vi "浊度电极校准.vi"() -> ()   [LabVIEW 2016, in "斯坦道多参数.lvlib"]
uses:
  <vilib>/Utility/miscctls.llb/LVPointTypeDef.ctl
  <vilib>/Analysis/NI_AALBase.lvlib
panel:
  out "第二点校准值":dbl
  out "第一点校准值":dbl
  in  "校准停止":bool
  in  "校准启动":bool
  in  "校准模式":enum16{"两点校准", "单点校准"}(ring)
  out "最小值":sgl format="%#.2f"
  out "最大值":sgl format="%#.2f"
  out "波形图表":sgl(graph) caption="历史曲线"
  out "mean":dbl caption="均值" format="%#.2f"
  out "standard deviation":dbl caption="标准差" format="%#.2f"
  out "变异系数":dbl format="%#.6f"
  out "测量值":dbl
  out "提示":string
  out "标液2":dbl
  out "标液1":dbl
  out "原始读取值":dbl caption="信号值"
  out "偏移值补偿":dbl
  out "电极斜率":dbl
  out "电极零点":dbl
  # "浊度电极设定"
  # "NTU"
  # "%"
  # "NTU"
  # "NTU"
  # "NTU"
  # "请选择校准模式:"
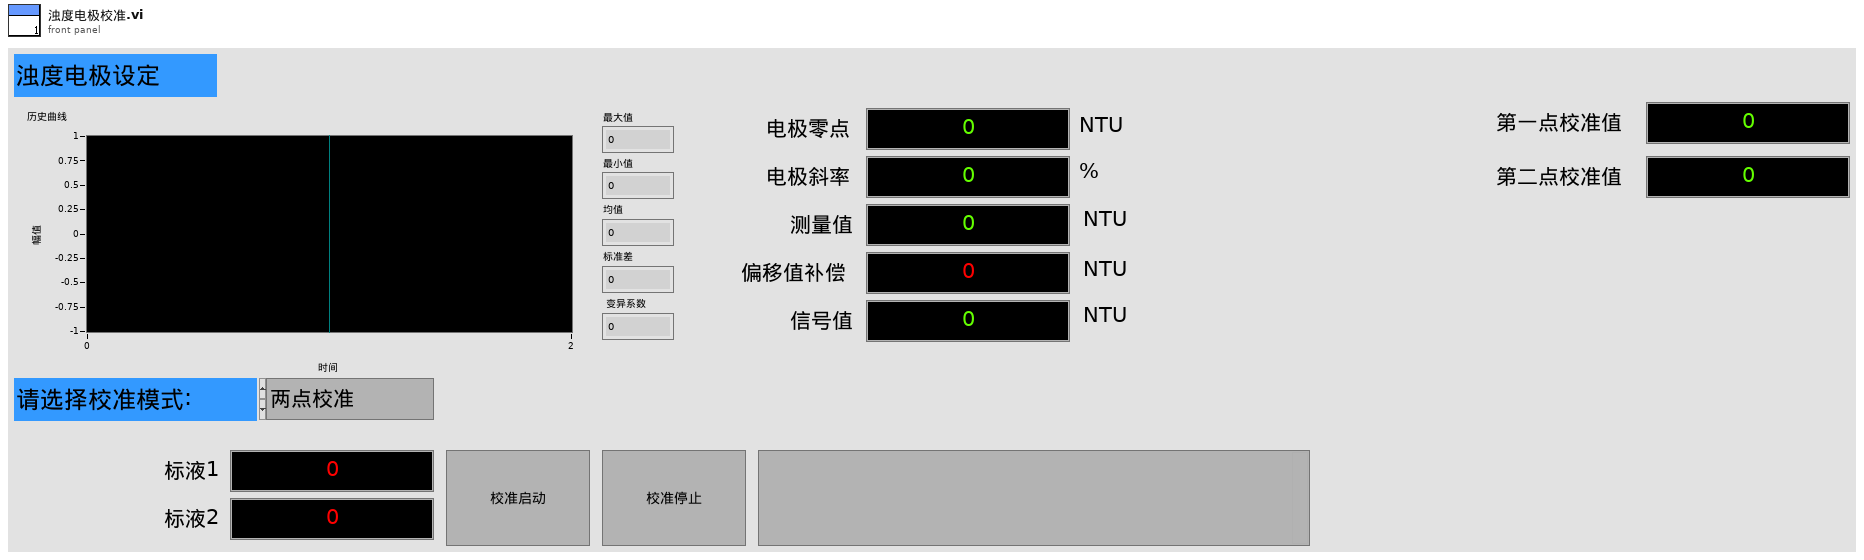
[diagram p1: front panel]
types:
  T1 = typedef "LVPointTypeDef.ctl" = cluster{"Horizontal":i16, "Vertical":i16}
  T2 = typedef "斯坦道多参数.lvlib/校准步骤.ctl" = enum16{"待机", "放置第一点标液", "第一点校准启动", "第一点校准写入", "第一点校准失败", "放置第二点标液", "第二点校准启动", "第二点校准写入", "第二点校准失败", "校准结果写入", "校准结束"}
  T3 = cluster{"电极状态标志":u16, "电极型号标志":u16, "浊度测量值":sgl, "温度测量值":sgl, "浊度信号值":sgl, "浊度偏移修正值":sgl, "温度偏移修正值":sgl, "手动温度补偿值":sgl, "浊度电极零点":sgl, "浊度电极斜率":sgl, "第1点标准值记录":sgl, "第1点信号值记录":sgl, "第1点温度值记录":sgl, "第2点标准值记录":sgl, "第2点信号值记录":sgl, "第2点温度值记录":sgl, "命令滤波设定":u16, "温度模式":enum16{"ATC", "MTC"}, "生产批次":u16, "电极序号":u16, "串口地址":u16, "串口波特率":enum16{"9600", "19200", "115200"}, "串口校验位":enum16{"NONE", "ODD", "EVEN"}, "串口停止位":enum16{"1bit", "2bit"}, "第一点标准值":sgl, "第二点标准值":sgl}
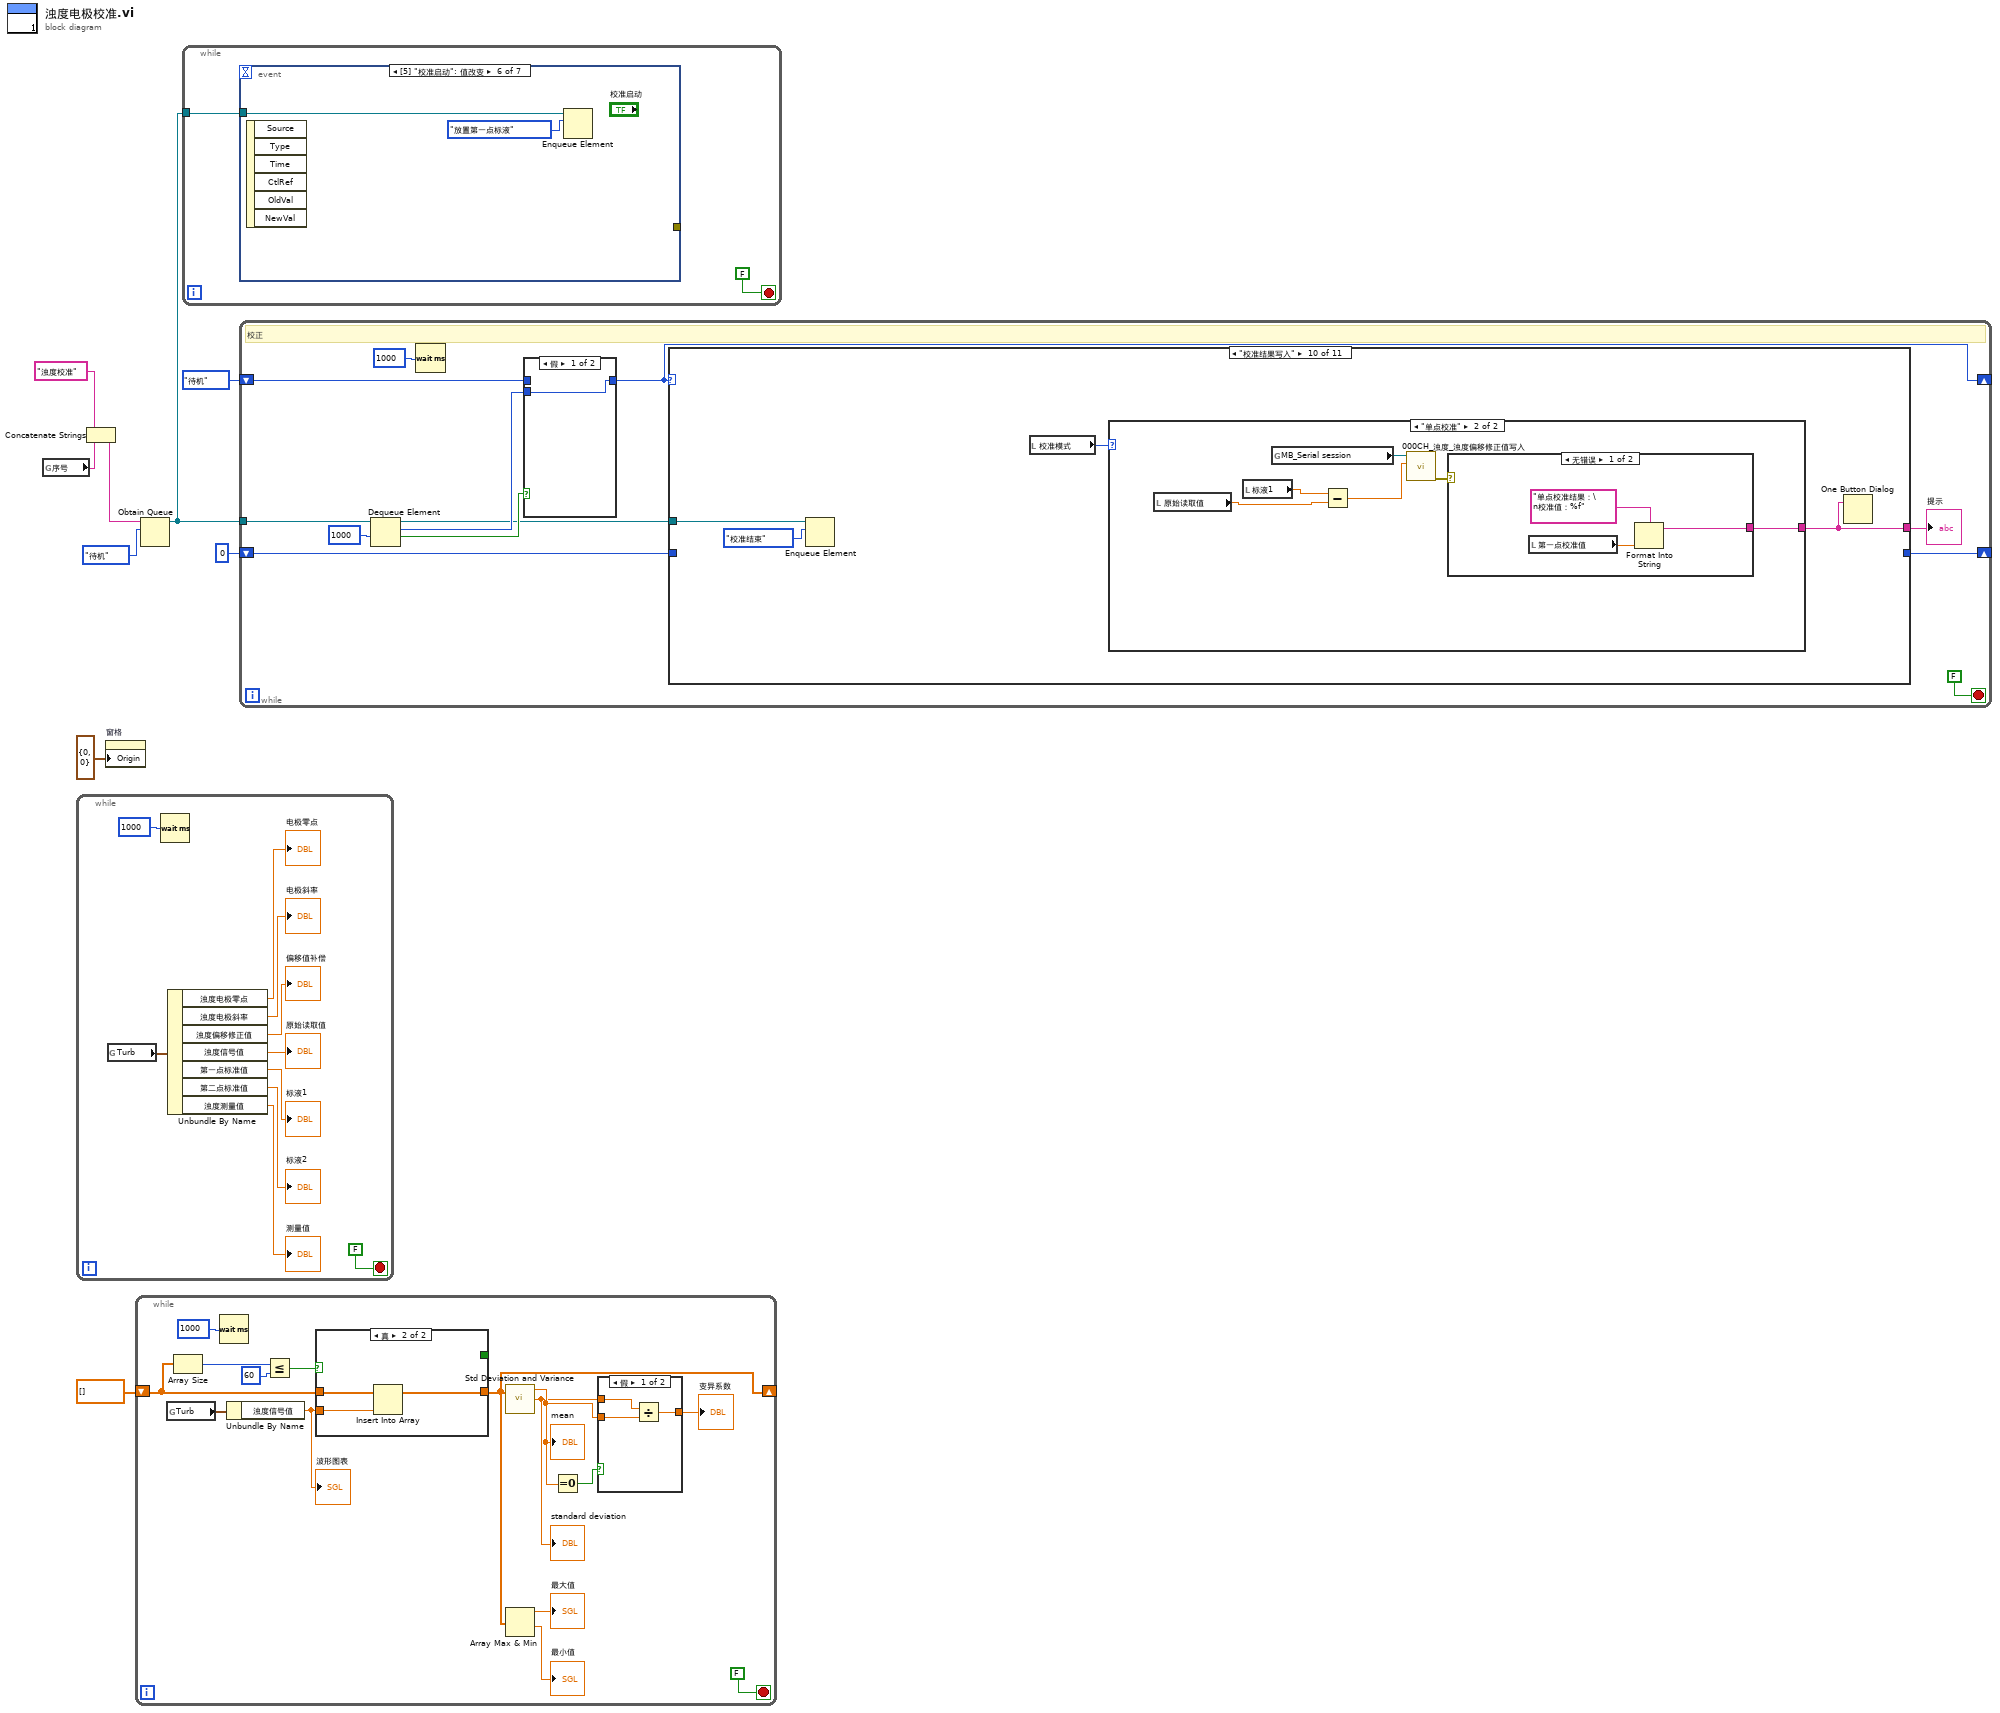
[diagram p0: block diagram]
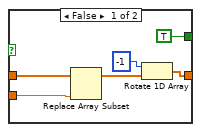
[diagram p3: hidden frame]
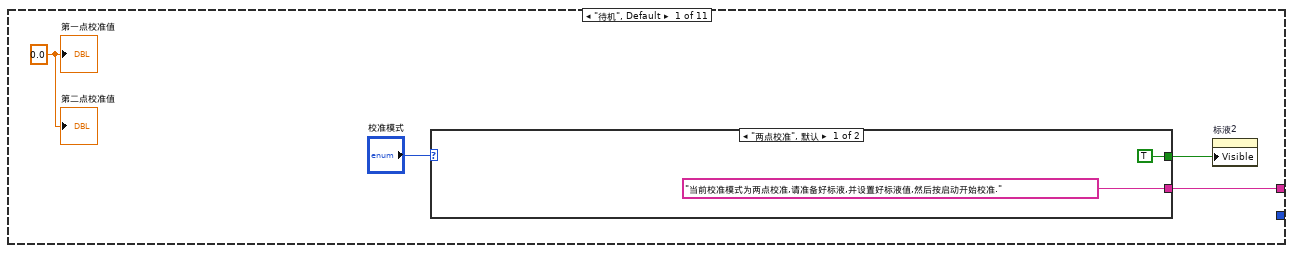
[diagram p5: hidden frame]
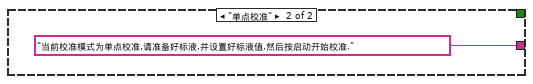
[diagram p6: hidden frame]
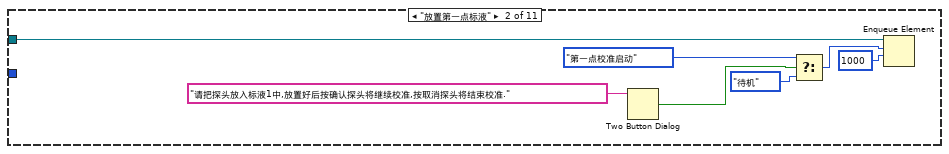
[diagram p7: hidden frame]
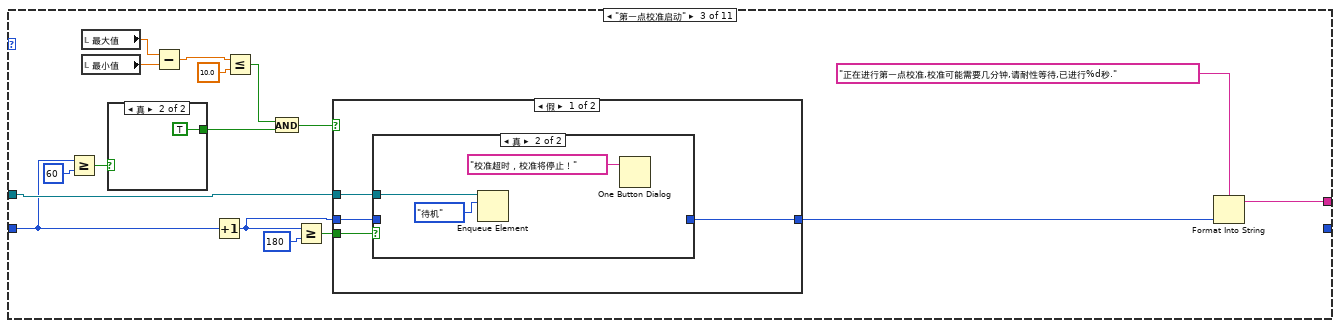
[diagram p8: hidden frame]
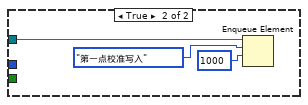
[diagram p10: hidden frame]
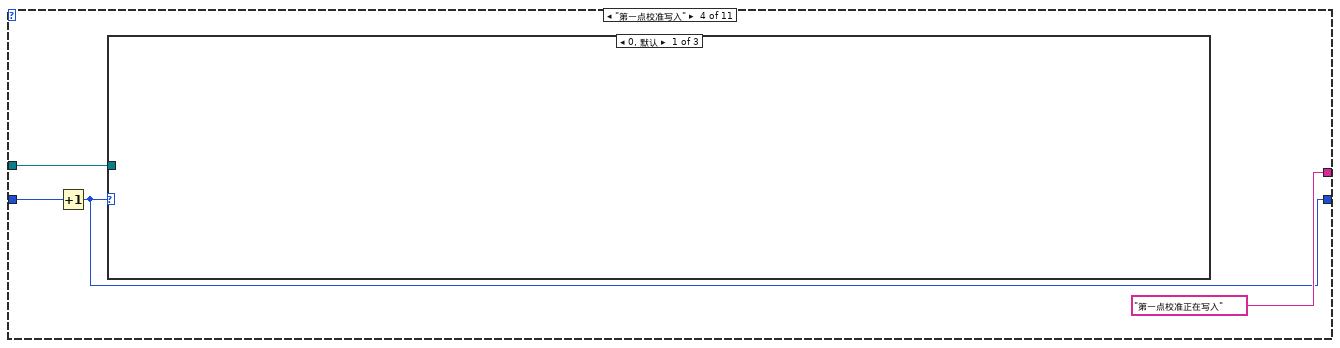
[diagram p12: hidden frame]
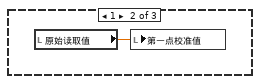
[diagram p13: hidden frame]
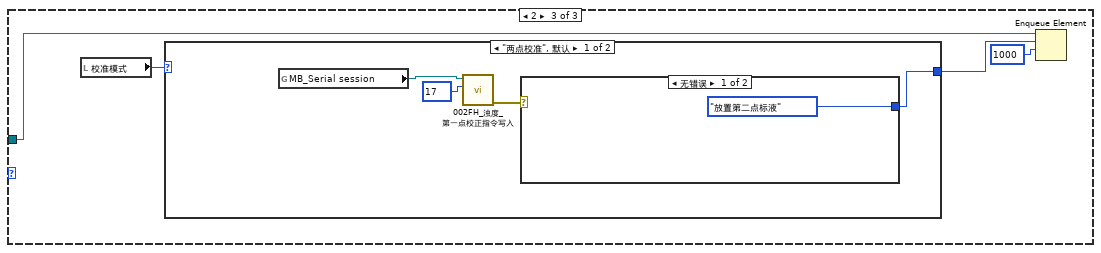
[diagram p14: hidden frame]
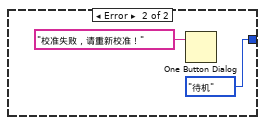
[diagram p15: hidden frame]
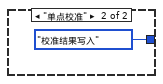
[diagram p16: hidden frame]
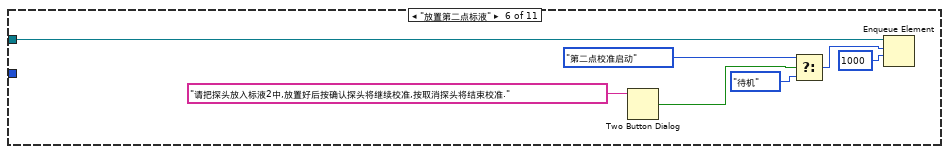
[diagram p18: hidden frame]
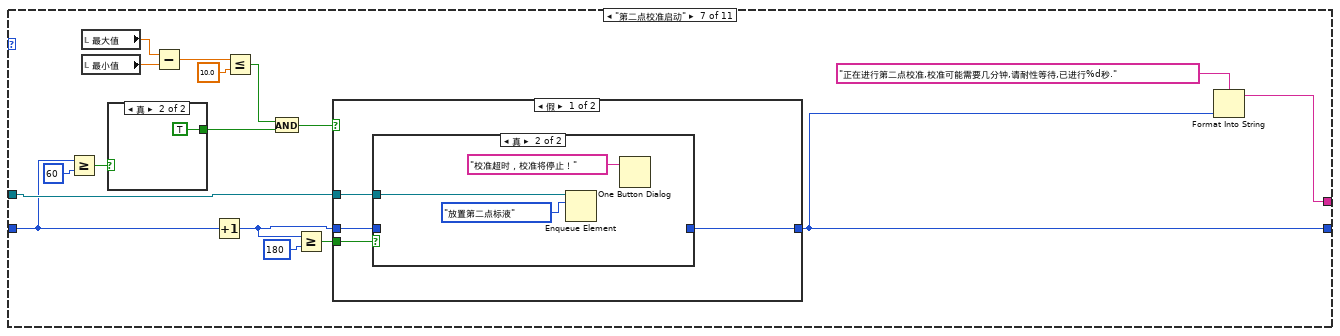
[diagram p19: hidden frame]
diagram:
  n1 = global read "多参数全局变量.vi" "序号"() -> (w1:string)
  n2 = while {
    stop <- FALSE stop-if-true
    n3 = global read "国弘过程全局变量.vi" "Turb"() -> (w17:T3)
    n4 = Wait (ms)(milliseconds to wait=u32 1000 ("等待时间（毫秒）")) -> ()  [unwired: 1 out]
    n5 = Unbundle By Name(w17) -> ("浊度电极零点"=→"电极零点":sgl, "浊度电极斜率"=→"电极斜率":sgl, "浊度偏移修正值"=→"偏移值补偿":sgl, "浊度信号值"=→"原始读取值":sgl, "第一点标准值"=→"标液1":sgl, "第二点标准值"=→"标液2":sgl, "浊度测量值"=→"测量值":sgl)
  }
  n6 = Concatenate Strings("浊度校准" ("名称（未命名）"), w1) -> (w2:string)
  n7 = property on="窗格" class="Pane"("Origin"=T1 {"Horizontal"=0, "Vertical"=0} ("原点")) -> ()  [unwired: 2 in, 2 out]
  n8 = while {
    shift-right: [w23] -> _
    shift-left: sgl[] [] -> [w30]
    stop <- FALSE stop-if-true
    n9 = global read "国弘过程全局变量.vi" "Turb"() -> (w24:T3)
    n10 = Array Size(array=w30) -> (size(s)=w32:i32)
    n11 = Wait (ms)(milliseconds to wait=u32 1000 ("等待时间（毫秒）")) -> ()  [unwired: 1 out]
    n12 = Unbundle By Name(w24) -> ("浊度信号值"=w20:sgl)
    "波形图表" <- w20
    n13 = Less Or Equal?(x=w32, y=60) -> (x <= y?=w31:bool)
    n14 = case shown="真" w31 {
      tunnel: w30 -> [w43 w46]
      tunnel: w20 -> [w41 w45]
      tunnel: [w39 w44] -> w23
      tunnel: [TRUE _] -> _
      frame False {
        n15 = Replace Array Subset(array=w43, new element=w41) -> (w42:sgl[])  [unwired: 1 in]
        n16 = Rotate 1D Array(1:w42, 2:-1 ("n")) -> (0:w39:sgl[])
      }
      frame True {
        n17 = Insert Into Array(array=w46, new element=w45) -> (w44:sgl[])  [unwired: 1 in]
      }
    }
    n18 = call <vilib>:"Std Deviation and Variance.vi"("X"=w23) -> ("mean"=w28:dbl, "standard deviation"=w27:dbl)  [unwired: 1 in, 1 out]
    "mean" <- w28
    "standard deviation" <- w27
    n19 = Array Max & Min(array=w23) -> (max value=→"最大值":sgl, min value=→"最小值":sgl)  [unwired: 2 out]
    n20 = Equal To 0?(x=w28) -> (x = 0?=w29:bool)
    n21 = case shown="假" w29 {
      tunnel: w27 -> [w37 _]
      tunnel: [w36 _] -> w26
      tunnel: w28 -> [w35 _]
      frame False {
        n22 = Divide(x=w37, y=w35) -> (x/y=w36:dbl)
      }
      frame True {
      }
    }
    "变异系数" <- w26
  }
  n23 = Obtain Queue(name (unnamed)=w2, element data type=校准步骤."待机" ("枚举")) -> (queue out=w4:refnum<queue>)  [unwired: 3 in, 2 out]
  n24 = while {
    tunnel: w4 -> [w47]
    stop <- FALSE stop-if-true
    n25 = event shown="[5] \"校准启动\": 值改变" {
      selector: _ -> [_ _ _ _ _ _ _]
      dyn-events: _ -> [_ _ _ _ _ _ _]
      timeout: _ -> [_ _ _ _ _ _ _]
      tunnel: [_ _ w54 w57 w61 _ _] -> _
      tunnel: w47 -> [_ _ _ _ _ w62 w64]
      event Timeout {
        n26 = event-data() -> ()  [unwired: 1 in, 3 out]
      }
      event "偏移值补偿", "标液1", "标液2": Mouse Down {
        n27 = event-data() -> ("CtlRef"=w49:refnum<vi>)  [unwired: 1 in, 7 out]
        n28 = property class="DigNum (严格)"(reference=w49) -> (reference out=w50:refnum<vi>, "Value"=w51:dbl)  [unwired: 1 in, 1 out]
        n29 = call "数字键盘.vi"("OldNumber"=w51) -> ("NewNumber"=w52:sgl)
        n30 = property class="DigNum (严格)"(reference=w50, "Val(Sgnl)"=w52) -> ()  [unwired: 1 in, 2 out]
      }
      event "偏移值补偿": Value Change {
        n31 = event-data() -> ("NewVal"=w55:dbl)  [unwired: 1 in, 5 out]
        n32 = global read "多参数全局变量.vi" "MB_Serial session"() -> (w53:refnum<class "MB_Master_Serial.lvclass">)
        n33 = call "000CH_浊度_浊度偏移修正值写入.vi"("数值"=w55, "MB_Serial session in"=w53) -> ("error out"=w54:errorcluster)  [unwired: 8 in, 1 out]
      }
      event "标液1": Value Change {
        n34 = event-data() -> ("NewVal"=w58:dbl)  [unwired: 1 in, 5 out]
        n35 = global read "多参数全局变量.vi" "MB_Serial session"() -> (w56:refnum<class "MB_Master_Serial.lvclass">)
        n36 = call "0030H_浊度_第一点标准值写入.vi"("数值"=w58, "MB_Serial session in"=w56) -> ("error out"=w57:errorcluster)  [unwired: 8 in, 1 out]
      }
      event "标液2": Value Change {
        n37 = event-data() -> ("NewVal"=w60:dbl)  [unwired: 1 in, 5 out]
        n38 = global read "多参数全局变量.vi" "MB_Serial session"() -> (w59:refnum<class "MB_Master_Serial.lvclass">)
        n39 = call "0033H_浊度_第二点标准值写入.vi"("数值"=w60, "MB_Serial session in"=w59) -> ("error out"=w61:errorcluster)  [unwired: 8 in, 1 out]
      }
      event "校准启动": Value Change {
        n40 = event-data() -> ()  [unwired: 1 in, 6 out]
        n41 = Enqueue Element(queue=w62, element=校准步骤."放置第一点标液" ("元素")) -> ()  [unwired: 2 in, 3 out]
      }
      event "校准停止": Value Change {
        n42 = event-data() -> ()  [unwired: 1 in, 6 out]
        n43 = Flush Queue(queue=w64) -> (queue out=w65:refnum<queue>)  [unwired: 1 in, 2 out]
        n44 = Enqueue Element(queue=w65, element=校准步骤."待机" ("元素"), timeout in ms (-1)=1000 ("超时毫秒(-1)")) -> ()  [unwired: 1 in, 3 out]
      }
    }
  }
  n45 = while "While循环" {
    shift-right: [w69] -> _
    shift-left: 校准步骤."待机" ("枚举") -> [w71]
    shift-right: [w68] -> _
    shift-left: 0 -> [w77]
    tunnel: w4 -> [w72]
    stop <- FALSE stop-if-true
    # "校正"
    n46 = Dequeue Element(queue=w72, timeout in ms (-1)=1000 ("超时毫秒(-1)")) -> (queue out=w70:refnum<queue>, element=w73:T2, timed out?=w74:bool)  [unwired: 1 in, 1 out]
    n47 = Wait (ms)(milliseconds to wait=u32 1000 ("等待时间（毫秒）")) -> ()  [unwired: 1 out]
    n48 = case shown="假" w74 {
      tunnel: w73 -> [w80 _]
      tunnel: [w80 w81] -> w69
      tunnel: w71 -> [_ w81]
      frame False {
      }
      frame True {
      }
    }
    n49 = case shown="\"校准结果写入\"" w69 {
      tunnel: [w83 _ w96 "第一点校准正在写入" ("提示") _ _ w151 "第二点校准正在写入" ("提示") "第二点校准失败" ("提示") w193 w224] -> w76
      tunnel: w77 -> [_ _ w98 w127 _ _ w152 w180 _ _ _]
      tunnel: [_ _ _ w125 _ _ w150 w178 _ _ _] -> w68
      tunnel: w70 -> [_ w89 w99 w126 _ w142 w153 w179 _ w195 _]
      frame "待机", Default {
        w85 = 0.0 ("第一点校准值")
        n50 = case shown="\"两点校准\", 默认" "校准模式" {
          tunnel: ["当前校准模式为两点校准,请准备好标液,并设置好标液值,然后按启动开始校准." ("提示") "当前校准模式为单点校准,请准备好标液,并设置好标液值,然后按启动开始校准." ("提示")] -> w83
          tunnel: [TRUE ("可见") _] -> w82
          frame "两点校准", Default {
          }
          frame "单点校准" {
          }
        }
        n51 = property on="标液2" class="DigNum (严格)"("Visible"=w82) -> ()  [unwired: 2 in, 2 out]
        "第一点校准值" <- w85
        "第二点校准值" <- w85
      }
      frame "放置第一点标液" {
        n52 = Two Button Dialog(message="请把探头放入标液1中,放置好后按确认探头将继续校准,按取消探头将结束校准." ("消息")) -> (T button?=w93:bool)  [unwired: 2 in]
        n53 = Select(t=校准步骤."第一点校准启动" ("元素"), s=w93, f=校准步骤."待机" ("元素")) -> (s? t:f=w90:T2)
        n54 = Enqueue Element(queue=w89, element=w90, timeout in ms (-1)=1000 ("超时毫秒(-1)")) -> ()  [unwired: 1 in, 3 out]
      }
      frame "第一点校准启动" {
        n55 = Greater Or Equal?(x=w98, y=60) -> (x >= y?=w105:bool)
        n56 = local read "最大值"() -> (w108:sgl)
        n57 = local read "最小值"() -> (w107:sgl)
        n58 = case shown="真" w105 {
          tunnel: [_ TRUE] -> w106
          frame False {
          }
          frame True {
          }
        }
        n59 = Subtract(x=w108, y=w107) -> (x-y=w109:sgl)
        n60 = Increment(x=w98) -> (x+1=w112:i32)
        n61 = Less Or Equal?(x=w109, y=10.0) -> (x <= y?=w102:bool)
        n62 = And(x=w102, y=w106) -> (x .and. y?=w110:bool)
        n63 = Greater Or Equal?(x=w112, y=180) -> (x >= y?=w111:bool)
        n64 = case shown="假" w110 {
          tunnel: w99 -> [w115 w123]
          tunnel: w111 -> [w116 _]
          tunnel: w112 -> [w114 _]
          tunnel: [w113 _] -> w97
          frame False {
            n65 = case shown="真" w116 {
              tunnel: w115 -> [_ w120]
              tunnel: w114 -> [w117 _]
              tunnel: [w117 _] -> w113
              frame False {
              }
              frame True {
                n66 = Enqueue Element(queue=w120, element=校准步骤."待机" ("元素")) -> ()  [unwired: 2 in, 3 out]
                n67 = One Button Dialog(message="校准超时，校准将停止！" ("消息")) -> ()  [unwired: 1 in, 1 out]
              }
            }
          }
          frame True {
            n68 = Enqueue Element(queue=w123, element=校准步骤."第一点校准写入" ("元素"), timeout in ms (-1)=1000 ("超时毫秒(-1)")) -> ()  [unwired: 1 in, 3 out]
          }
        }
        n69 = Format Into String(format string="正在进行第一点校准,校准可能需要几分钟,请耐性等待,已进行%d秒." ("格式字符串"), w97) -> (resulting string=w96:string)  [unwired: 2 in, 1 out]
      }
      frame "第一点校准写入" {
        n70 = Increment(x=w127) -> (x+1=w125:i32)
        n71 = case shown="0, 默认" w125 {
          tunnel: w126 -> [_ _ w133]
          frame 0, Default {
          }
          frame 1 {
            n72 = local read "原始读取值"() -> (w129:dbl)
            n73 = local write "第一点校准值"(w129) -> ()
          }
          frame 2 {
            n74 = local read "校准模式"() -> (w132:enum16{"两点校准", "单点校准"})
            n75 = case shown="\"两点校准\", 默认" w132 {
              tunnel: [w134 校准步骤."校准结果写入" ("元素")] -> w131
              frame "两点校准", Default {
                n76 = global read "多参数全局变量.vi" "MB_Serial session"() -> (w137:refnum<class "MB_Master_Serial.lvclass">)
                n77 = call "002FH_浊度_第一点校正指令写入.vi"("数值"=u16 17, "MB_Serial session in"=w137) -> ("error out"=w135:errorcluster)  [unwired: 8 in, 1 out]
                n78 = case shown="无错误" w135 {
                  tunnel: [校准步骤."放置第二点标液" ("元素") 校准步骤."待机" ("元素")] -> w134
                  frame No Error {
                  }
                  frame Error {
                    n79 = One Button Dialog(message="校准失败，请重新校准！" ("消息")) -> ()  [unwired: 1 in, 1 out]
                  }
                }
              }
              frame "单点校准" {
              }
            }
            n80 = Enqueue Element(queue=w133, element=w131, timeout in ms (-1)=1000 ("超时毫秒(-1)")) -> ()  [unwired: 1 in, 3 out]
          }
        }
      }
      frame "第一点校准失败" {
      }
      frame "放置第二点标液" {
        n81 = Two Button Dialog(message="请把探头放入标液2中,放置好后按确认探头将继续校准,按取消探头将结束校准." ("消息")) -> (T button?=w146:bool)  [unwired: 2 in]
        n82 = Select(t=校准步骤."第二点校准启动" ("元素"), s=w146, f=校准步骤."待机" ("元素")) -> (s? t:f=w143:T2)
        n83 = Enqueue Element(queue=w142, element=w143, timeout in ms (-1)=1000 ("超时毫秒(-1)")) -> ()  [unwired: 1 in, 3 out]
      }
      frame "第二点校准启动" {
        n84 = Greater Or Equal?(x=w152, y=60) -> (x >= y?=w158:bool)
        n85 = local read "最大值"() -> (w161:sgl)
        n86 = local read "最小值"() -> (w160:sgl)
        n87 = case shown="真" w158 {
          tunnel: [_ TRUE] -> w159
          frame False {
          }
          frame True {
          }
        }
        n88 = Subtract(x=w161, y=w160) -> (x-y=w162:sgl)
        n89 = Increment(x=w152) -> (x+1=w165:i32)
        n90 = Less Or Equal?(x=w162, y=10.0) -> (x <= y?=w155:bool)
        n91 = And(x=w155, y=w159) -> (x .and. y?=w163:bool)
        n92 = Greater Or Equal?(x=w165, y=180) -> (x >= y?=w164:bool)
        n93 = case shown="假" w163 {
          tunnel: w153 -> [w168 w176]
          tunnel: w164 -> [w169 _]
          tunnel: w165 -> [w167 _]
          tunnel: [w166 _] -> w150
          frame False {
            n94 = case shown="真" w169 {
              tunnel: w168 -> [_ w173]
              tunnel: w167 -> [w170 _]
              tunnel: [w170 _] -> w166
              frame False {
              }
              frame True {
                n95 = Enqueue Element(queue=w173, element=校准步骤."放置第二点标液" ("元素")) -> ()  [unwired: 2 in, 3 out]
                n96 = One Button Dialog(message="校准超时，校准将停止！" ("消息")) -> ()  [unwired: 1 in, 1 out]
              }
            }
          }
          frame True {
            n97 = Enqueue Element(queue=w176, element=校准步骤."第二点校准写入" ("元素"), timeout in ms (-1)=1000 ("超时毫秒(-1)")) -> ()  [unwired: 1 in, 3 out]
          }
        }
        n98 = Format Into String(format string="正在进行第二点校准,校准可能需要几分钟,请耐性等待,已进行%d秒." ("格式字符串"), w150) -> (resulting string=w151:string)  [unwired: 2 in, 1 out]
      }
      frame "第二点校准写入" {
        n99 = Increment(x=w180) -> (x+1=w178:i32)
        n100 = case shown="1" w178 {
          tunnel: w179 -> [_ _ w188]
          frame 0, Default {
          }
          frame 1 {
            n101 = local read "原始读取值"() -> (w182:dbl)
            n102 = local write "第二点校准值"(w182) -> ()
          }
          frame 2 {
            n103 = global read "多参数全局变量.vi" "MB_Serial session"() -> (w183:refnum<class "MB_Master_Serial.lvclass">)
            n104 = call "0032H_浊度_第二点校正指令写入.vi"("数值"=u16 33, "MB_Serial session in"=w183) -> ("error out"=w184:errorcluster)  [unwired: 8 in, 1 out]
            n105 = case shown="无错误" w184 {
              tunnel: [校准步骤."校准结果写入" ("元素") 校准步骤."放置第二点标液" ("元素")] -> w186
              frame No Error {
              }
              frame Error {
                n106 = One Button Dialog(message="校准失败，请重新校准！" ("消息")) -> ()  [unwired: 1 in, 1 out]
              }
            }
            n107 = Enqueue Element(queue=w188, element=w186, timeout in ms (-1)=1000 ("超时毫秒(-1)")) -> ()  [unwired: 1 in, 3 out]
          }
        }
      }
      frame "第二点校准失败" {
      }
      frame "校准结果写入" {
        n108 = Enqueue Element(queue=w195, element=校准步骤."校准结束" ("元素")) -> ()  [unwired: 2 in, 3 out]
        n109 = local read "校准模式"() -> (w194:enum16{"两点校准", "单点校准"})
        n110 = case shown="\"单点校准\"" w194 {
          tunnel: [w199 w218] -> w193
          frame "两点校准", Default {
            n111 = global read "国弘过程全局变量.vi" "Turb"() -> (w198:T3)
            n112 = Unbundle By Name(w198) -> ("电极状态标志"=w197:u16)
            n113 = case shown="2" w197 {
              selector: w197 -> [w201 _ w210]
              tunnel: [w200 w205 w209] -> w199
              frame 0, Default {
                n114 = case shown="0, 默认" w201 {
                  tunnel: ["校正未正常启动，请重新校正" "第一点校准通过" "第二点校准通过"] -> w200
                  frame 0, Default {
                  }
                  frame 1 {
                  }
                  frame 2 {
                  }
                }
              }
              frame 2 {
                n115 = local read "第一点校准值"() -> (w207:dbl)
                n116 = local read "第二点校准值"() -> (w208:dbl)
                n117 = Format Into String(format string="两点校准结果：\n第一点校准值：%f\n第二点校准值：%f" ("提示"), w207, w208) -> (resulting string=w205:string)  [unwired: 2 in, 1 out]
              }
              frame 3, 4 {
                n118 = case shown="4" w210 {
                  tunnel: ["校正失败，电极零点超出范围" "校正失败，电极斜率超出范围"] -> w209
                  frame 3, Default {
                  }
                  frame 4 {
                  }
                }
              }
            }
          }
          frame "单点校准" {
            n119 = local read "原始读取值"() -> (w217:dbl)
            n120 = local read "标液1"() -> (w216:dbl)
            n121 = global read "多参数全局变量.vi" "MB_Serial session"() -> (w215:refnum<class "MB_Master_Serial.lvclass">)
            n122 = Subtract(x=w216, y=w217) -> (x-y=w213:dbl)
            n123 = call "000CH_浊度_浊度偏移修正值写入.vi"("数值"=w213, "MB_Serial session in"=w215) -> ("error out"=w214:errorcluster)  [unwired: 8 in, 1 out]
            n124 = case shown="无错误" w214 {
              tunnel: [w219 "校准失败"] -> w218
              frame No Error {
                n125 = local read "第一点校准值"() -> (w221:dbl)
                n126 = Format Into String(format string="单点校准结果：\n校准值：%f" ("提示"), w221) -> (resulting string=w219:string)  [unwired: 2 in, 1 out]
              }
              frame Error {
                n127 = One Button Dialog(message="校准失败，请重新校准！" ("消息")) -> ()  [unwired: 1 in, 1 out]
              }
            }
          }
        }
        n128 = One Button Dialog(message=w193) -> ()  [unwired: 1 in, 1 out]
      }
      frame "校准结束" {
        n129 = local read "提示"() -> (w224:string)
      }
    }
    "提示" <- w76
  }
